vi "dvp Vi Get Accelerate Sel.vi"(10 "pAccelerateSel":u32, 11 "handle":u32) -> (2 "pAccelerateSel out":u32, 3 "function return":u32(ring))   [LabVIEW 2018, in "LabViewDVPCamera.lvlib"]
doc: "LabviewDvp2Api dvpStatus dvpViGetAccelerateSel(dvpHandle handle, dvpUint32 *pAccelerateSel);"
uses:
  LabViewDVPCamera.lvlib
  LabViewDVPCamera/LabViewDVPCamera.dll
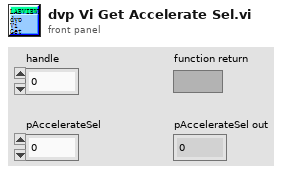
[diagram p1: front panel]
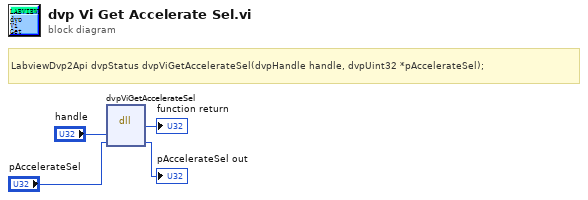
[diagram p0: block diagram]
diagram:
  # "LabviewDvp2Api dvpStatus dvpViGetAccelerateSel(dvpHandle handle, dvpUint32 *pAccelerateSel);"
  n1 = dll-call lib="C:/Program Files (x86)/DVP2 Labview cn 64/Sample/LabViewDVPCamera/LabViewDVPCamera.*" fn="dvpViGetAccelerateSel"("handle"="handle", "pAccelerateSel"="pAccelerateSel") -> (→"function return":u32, "pAccelerateSel"=→"pAccelerateSel out":u32)  [unwired: 4 in, 2 out]
